vi "Send Message Module Synchronous.vi"(7 "priority (normal)":T1, 8 "Error In":errorcluster, 9 "Data":variant, 10 "Message":string, 11 "Target ModuleName In":T2=enum."Controller") -> (0 "error in (no error)":errorcluster, 3 "Message Response":variant)   [LabVIEW 2019, in "Architecture.lvlib"]
doc: "This method is used to send a synchronous message to a target module. It generates a user event that will be handled by target module's event structure. Once the user event is generated, this method waits on a notification from the destination module as a response."
uses:
  Architecture.lvlib
  Typedefs/Enum_Module_Name.ctl
  <vilib>/event_ctls.llb/usereventprio.ctl
  Typedefs/Module References.ctl
  Typedefs/Message.ctl
  Typedefs/FGV Ref. Modules Function.ctl
panel:
  out "timed out?":bool
  in  "timeout in ms (-1)":i32
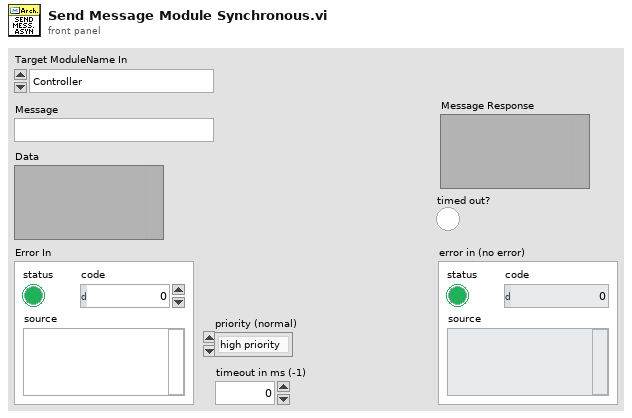
[diagram p1: front panel]
types:
  T1 = typedef "usereventprio.ctl" = enum32{"high priority", "normal priority"}
  T2 = typedef "Architecture.lvlib/Enum_Module_Name.ctl" = enum16{"Configuration", "Error_Handler", "Log", "Database", "Controller", "User Console", "Display Console", "Sensor Interface"}
  T3 = typedef "Architecture.lvlib/Message.ctl" = cluster{"Message":string, "Data":variant, "syn":bool}
  T4 = typedef "Architecture.lvlib/FGV Ref. Modules Function.ctl" = enum16{"Init ", "Add Module", "Get Module", "Get All", "Add Asynchronous Run Ref", "Dispose"}
  T5 = typedef "Architecture.lvlib/Module References.ctl" = cluster{"ModuleName":T2, "Queue":refnum<queue>, "user event":refnum<user-event>, "VI Refnum":refnum<vi>, "ShowFP":bool, "StatesTracking Enabled":bool}
  T6 = cluster{"Data":variant, "notifier out":refnum<notifier>}
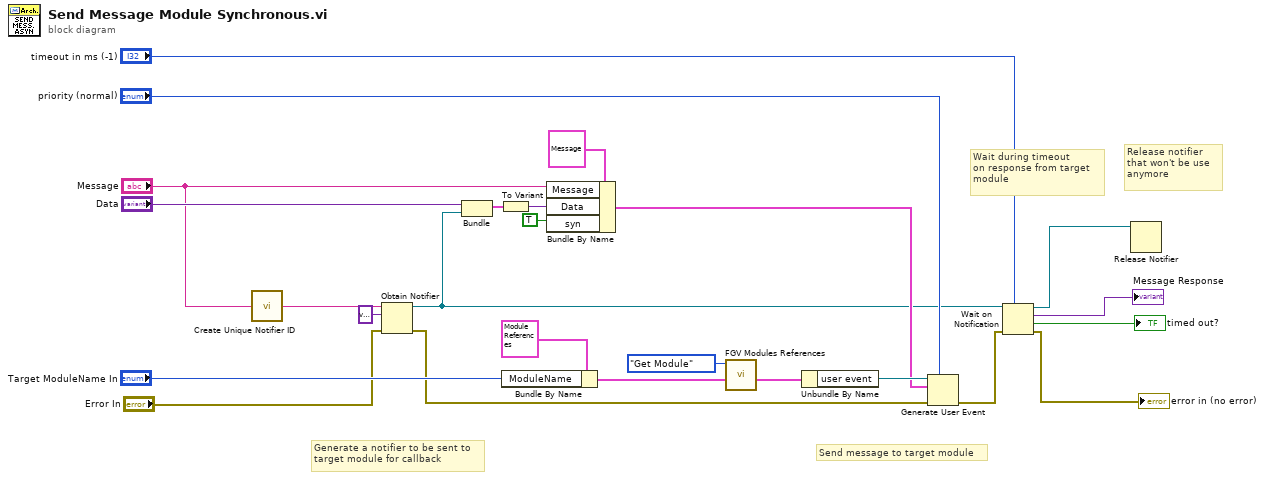
[diagram p0: block diagram]
diagram:
  # "Release notifier \nthat won't be use \nanymore"
  # "Send message to target module"
  # "Wait during timeout \non response from target \nmodule"
  # "Generate a notifier to be sent to \ntarget module for callback"
  n1 = call "Create Unique Notifier ID.vi"("Message Name"="Message") -> ("ID Out"=w12:string)
  n2 = Obtain Notifier(name (unnamed)=w12, notification data type=variant ("element data type"), error in (no error)="Error In") -> (notifier out=w2:refnum<notifier>, error out=w11:errorcluster)  [unwired: 1 in, 1 out]
  n3 = Bundle("Data"="Data", "notifier out"=w2) -> (w3:T6)  [unwired: 1 in]
  n4 = To Variant(anything=w3) -> (Variant=w1:variant)
  n5 = Bundle By Name(cluster=T5 {"ModuleName"=enum."Controller", "Queue"=refnum, "user event"=refnum, "VI Refnum"=refnum, "ShowFP"=FALSE, "StatesTracking Enabled"=FALSE} ("Module_Refs"), "ModuleName"="Target ModuleName In") -> (w23:T5)
  n6 = Bundle By Name(cluster=T3 {"Message"="", "Data"=variant, "syn"=FALSE} ("event data"), "Message"="Message", "Data"=w1, "syn"=TRUE) -> (w19:T3)
  n7 = call "FGV Modules References.vi"("Module_Refs"=w23, "FGV Ref. Function In"=FGV_Ref._Modules_Function."Get Module") -> ("Module_Ref Out"=w21:T5)  [unwired: 7 in, 2 out]
  n8 = Unbundle By Name(w21) -> ("user event"=w20:refnum<user-event>)
  n9 = Generate User Event(priority (normal)="priority (normal)", user event=w20, event data cluster=w19, error in=w11) -> (error out=w16:errorcluster)  [unwired: 1 out]
  n10 = Wait on Notification(notifier=w2, timeout in ms (-1)="timeout in ms (-1)", error in (no error)=w16) -> (notifier out=w4:refnum<notifier>, notification=→"Message Response":variant, timed out?=→"timed out?":bool, error out=→"error in (no error)":errorcluster)  [unwired: 1 in]
  n11 = Release Notifier(notifier=w4) -> ()  [unwired: 2 in, 3 out]
